vi "Initialize Attributes.vi"(8 "error in (no error)":errorcluster, 10 "Attribute Data":variant, 11 "CS++DCPwr in":refnum<class "CS++DCPwr.lvclass">) -> (0 "error out":errorcluster, 2 "Found?":bool, 3 "CS++DCPwr out":refnum<class "CS++DCPwr.lvclass">)   [LabVIEW 2013, in "CS++DCPwr.lvlib" / "CS++DCPwr.lvclass"]
doc: "Initialize object attribute.\n\nUnique resources should be allocated elsewhere!"
uses:
  CS++DCPwr.lvclass
  Core/Actors/CS++DeviceActor/CS++DeviceActor.lvclass
  Core/Actors/CS++BaseActor/CS++BaseActor.lvclass/CS++BaseActor.ctl
  Core/Classes/CS++BaseClasses/Factory/CS++Factory.lvclass
  CS++DCPwr.lvclass/CS++DCPwr.ctl
  Core/Actors/CS++BaseActor/CS++BaseActor.lvclass
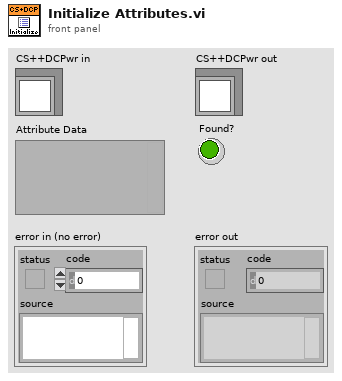
[diagram p1: front panel]
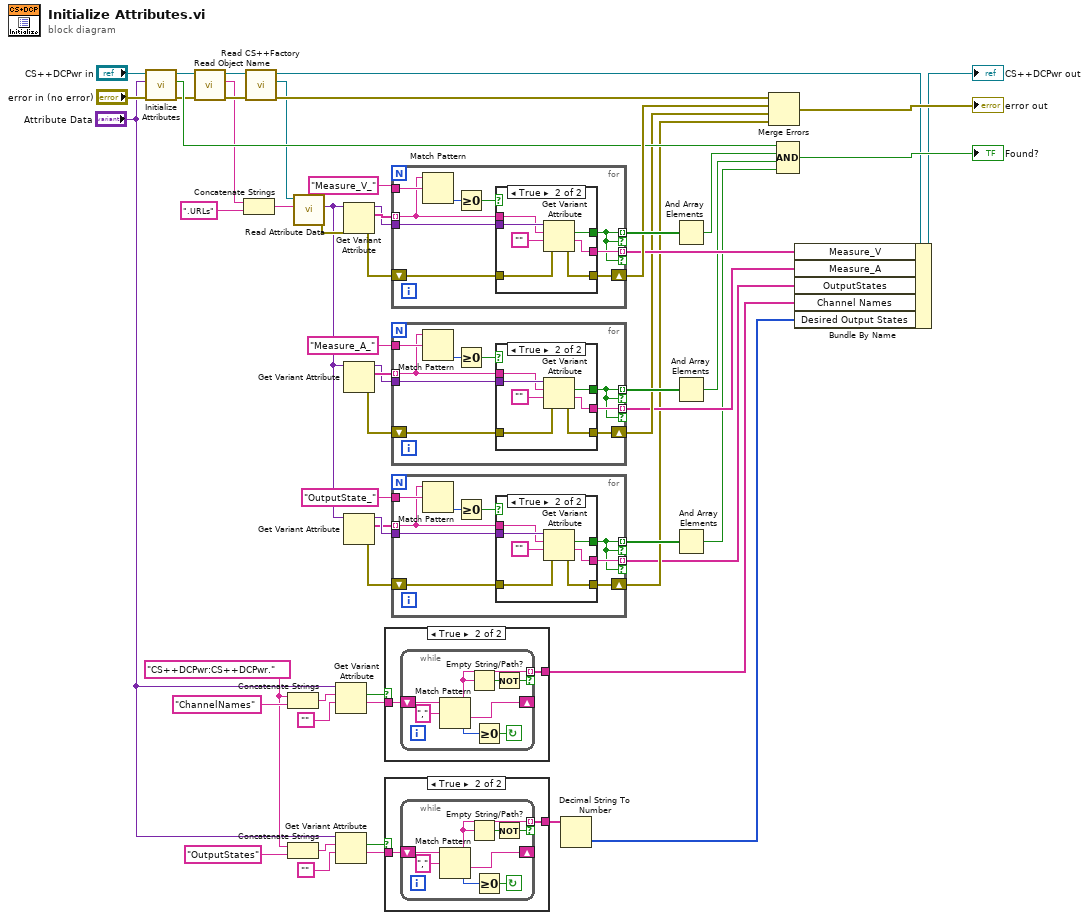
[diagram p0: block diagram]
diagram:
  w4 = "CS++DCPwr:CS++DCPwr."
  n1 = call-parent "Initialize Attributes.vi"("error in (no error)"="error in (no error)", "Attribute Data"="Attribute Data", "CS++DeviceActor in"="CS++DCPwr in") -> ("error out"=w46:errorcluster, "Found?"=w48:bool, "CS++DeviceActor out"=w47:refnum<class "CS++DCPwr.lvclass">)  [unwired: 6 in]
  n2 = call "Read Object Name.vi"("error in (no error)"=w46, "CS++BaseActor in"=w47) -> ("error out"=w50:errorcluster, "Object Name"=w33:string, "CS++BaseActor out"=w53:refnum<class "CS++DCPwr.lvclass">)  [unwired: 7 in]
  n3 = Concatenate Strings(w33, ".URLs" ("string")) -> (w54:string)
  n4 = call "Read CS++Factory.vi"("error in (no error)"=w50, "CS++BaseActor in"=w53) -> ("error out"=w49:errorcluster, "CS++Factory"=w29:refnum<class "CS++Factory.lvclass">, "CS++BaseActor out"=w39:refnum<class "CS++DCPwr.lvclass">)  [unwired: 7 in]
  n5 = Concatenate Strings(w4, "ChannelNames" ("string")) -> (w27:string)
  n6 = Concatenate Strings(w4, "OutputStates" ("string")) -> (w6:string)
  n7 = call-dynamic "Read Attribute Data.vi"("Object Name"=w54, "CS++Factory in"=w29) -> ("error out"=w43:errorcluster, "Attribute Data"=w14:variant)  [unwired: 7 in, 1 out]
  n8 = Get Variant Attribute(Variant="Attribute Data", name=w27, default value (empty Variant)="") -> (found=w24:bool, value=w25:string)  [unwired: 1 in, 2 out]
  n9 = Get Variant Attribute(Variant="Attribute Data", name=w6, default value (empty Variant)="") -> (found=w9:bool, value=w8:string)  [unwired: 1 in, 2 out]
  n10 = Get Variant Attribute(Variant=w14, error in=w43) -> (duplicate Variant=w19:variant, names=w41:string[], error out=w42:errorcluster)  [unwired: 2 in, 1 out]
  n11 = Get Variant Attribute(Variant=w14) -> (duplicate Variant=w20:variant, names=w36:string[], error out=w35:errorcluster)  [unwired: 3 in, 1 out]
  n12 = Get Variant Attribute(Variant=w14) -> (duplicate Variant=w18:variant, names=w15:string[], error out=w16:errorcluster)  [unwired: 3 in, 1 out]
  n13 = case shown="True" w24 {
    tunnel: w25 -> [_ w59]
    tunnel: [_ w58] -> w23
    frame False {
    }
    frame True {
      n14 = while {
        shift-right: [w65] -> _
        shift-left: w59 -> [w67]
        tunnel: [w61] -> w58 mode=indexing if=w60
        stop <- w63 continue-if-true
        n15 = Match Pattern(string=w67, regular expression=",") -> (before substring=w61:string, after substring=w65:string, offset past match=w64:i32)  [unwired: 1 in, 1 out]
        n16 = Empty String/Path?(string/path=w61) -> (empty?=w62:bool)
        n17 = Greater Or Equal To 0?(x=w64) -> (x >= 0?=w63:bool)
        n18 = Not(x=w62) -> (.not. x?=w60:bool)
      }
    }
  }
  n19 = case shown="True" w9 {
    tunnel: w8 -> [_ w69]
    tunnel: [_ w68] -> w3
    frame False {
    }
    frame True {
      n20 = while {
        shift-right: [w75] -> _
        shift-left: w69 -> [w77]
        tunnel: [w71] -> w68 mode=indexing if=w70
        stop <- w73 continue-if-true
        n21 = Match Pattern(string=w77, regular expression=",") -> (before substring=w71:string, after substring=w75:string, offset past match=w74:i32)  [unwired: 1 in, 1 out]
        n22 = Empty String/Path?(string/path=w71) -> (empty?=w72:bool)
        n23 = Greater Or Equal To 0?(x=w74) -> (x >= 0?=w73:bool)
        n24 = Not(x=w72) -> (.not. x?=w70:bool)
      }
    }
  }
  n25 = for {
    tunnel: [w78] -> w52 mode=indexing if=w78
    tunnel: w19 -> [w84]
    shift-right: [w86] -> w51
    shift-left: w42 -> [w85]
    tunnel: w41 -> [w82] mode=indexing
    tunnel: "Measure_V_" ("string") -> [w83]
    tunnel: [w79] -> w37 mode=indexing if=w78
    n26 = Match Pattern(string=w82, regular expression=w83) -> (offset past match=w81:i32)  [unwired: 1 in, 3 out]
    n27 = Greater Or Equal To 0?(x=w81) -> (x >= 0?=w80:bool)
    n28 = case shown="True" w80 {
      tunnel: [_ w93] -> w78
      tunnel: [w87 w92] -> w86
      tunnel: w85 -> [w87 w91]
      tunnel: w84 -> [_ w90]
      tunnel: w82 -> [_ w89]
      tunnel: [_ w88] -> w79
      frame False {
      }
      frame True {
        n29 = Get Variant Attribute(Variant=w90, name=w89, default value (empty Variant)="", error in=w91) -> (found=w93:bool, value=w88:string, error out=w92:errorcluster)  [unwired: 1 out]
      }
    }
  }
  n30 = for {
    tunnel: [w95] -> w34 mode=indexing if=w95
    tunnel: w20 -> [w101]
    shift-right: [w103] -> w32
    shift-left: w35 -> [w102]
    tunnel: w36 -> [w99] mode=indexing
    tunnel: "Measure_A_" ("string") -> [w100]
    tunnel: [w96] -> w30 mode=indexing if=w95
    n31 = Match Pattern(string=w99, regular expression=w100) -> (offset past match=w98:i32)  [unwired: 1 in, 3 out]
    n32 = Greater Or Equal To 0?(x=w98) -> (x >= 0?=w97:bool)
    n33 = case shown="True" w97 {
      tunnel: [_ w110] -> w95
      tunnel: [w104 w109] -> w103
      tunnel: w102 -> [w104 w108]
      tunnel: w101 -> [_ w107]
      tunnel: w99 -> [_ w106]
      tunnel: [_ w105] -> w96
      frame False {
      }
      frame True {
        n34 = Get Variant Attribute(Variant=w107, name=w106, default value (empty Variant)="", error in=w108) -> (found=w110:bool, value=w105:string, error out=w109:errorcluster)  [unwired: 1 out]
      }
    }
  }
  n35 = for {
    tunnel: [w112] -> w13 mode=indexing if=w112
    tunnel: w18 -> [w118]
    shift-right: [w120] -> w11
    shift-left: w16 -> [w119]
    tunnel: w15 -> [w116] mode=indexing
    tunnel: "OutputState_" ("string") -> [w117]
    tunnel: [w113] -> w10 mode=indexing if=w112
    n36 = Match Pattern(string=w116, regular expression=w117) -> (offset past match=w115:i32)  [unwired: 1 in, 3 out]
    n37 = Greater Or Equal To 0?(x=w115) -> (x >= 0?=w114:bool)
    n38 = case shown="True" w114 {
      tunnel: [_ w127] -> w112
      tunnel: [w121 w126] -> w120
      tunnel: w119 -> [w121 w125]
      tunnel: w118 -> [_ w124]
      tunnel: w116 -> [_ w123]
      tunnel: [_ w122] -> w113
      frame False {
      }
      frame True {
        n39 = Get Variant Attribute(Variant=w124, name=w123, default value (empty Variant)="", error in=w125) -> (found=w127:bool, value=w122:string, error out=w126:errorcluster)  [unwired: 1 out]
      }
    }
  }
  n40 = Decimal String To Number(string=w3) -> (number=w1:i32[])  [unwired: 2 in, 1 out]
  n41 = And Array Elements(Boolean array=w52) -> (logical AND=w40:bool)
  n42 = And Array Elements(Boolean array=w34) -> (logical AND=w31:bool)
  n43 = And Array Elements(Boolean array=w13) -> (logical AND=w12:bool)
  n44 = Merge Errors(w49, w51, w32, w11) -> (→"error out":errorcluster)
  n45 = Compound Arithmetic op=AND(w48, w40, w31, w12) -> (→"Found?":bool)
  n46 = Bundle By Name(cluster=w39, "Measure_V"=w37, "Measure_A"=w30, "OutputStates"=w10, "Channel Names"=w23, "Desired Output States"=w1) -> (→"CS++DCPwr out":refnum<class "CS++DCPwr.lvclass">)
